vi "Write_To_XML_File.vi"(11 "2D-Array":dbl[][](array[numeric])) -> ()   [LabVIEW 2024]
uses:
  <vilib>/Utility/xml.llb/Read From XML File(string).vi
  <vilib>/Utility/xml.llb/Write to XML File(string).vi
panel:
  in  "Write to XML":bool
  in  "stop":bool
  out "XML Output":string
  out "XML File Path":path
  # "Suppose the 2 D Array is updated at different time. As it is not automated in this VI enter some values\nin the 2D array and press the Write to XML button. Check the output.!!"
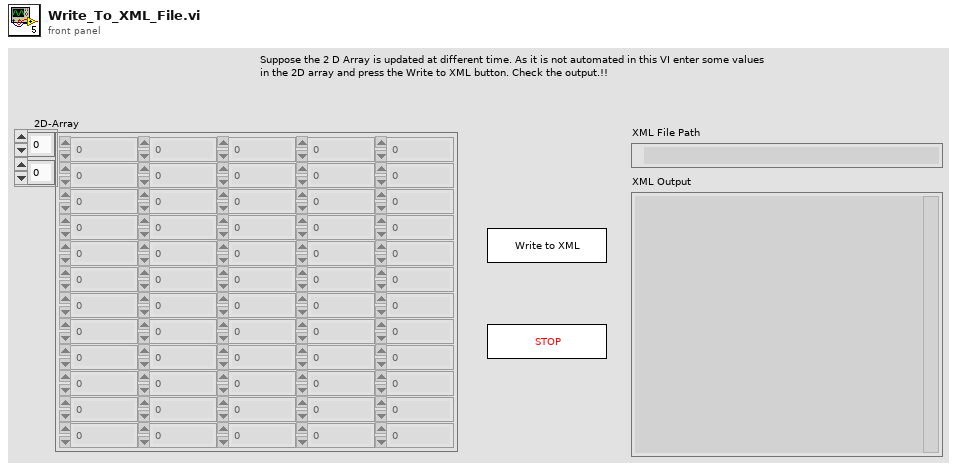
[diagram p1: front panel]
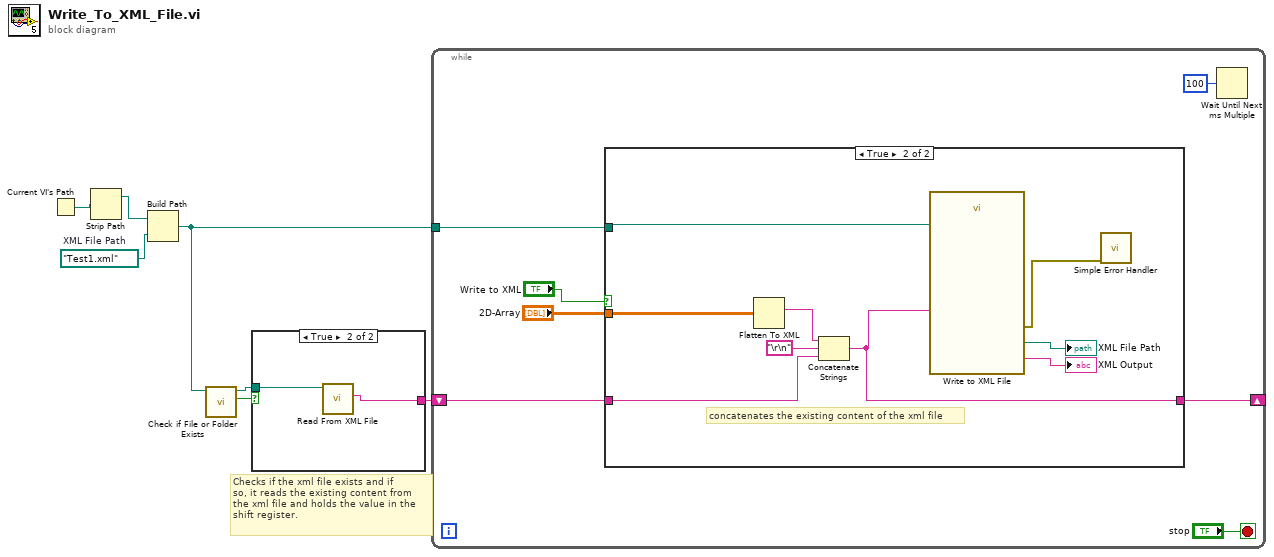
[diagram p0: block diagram]
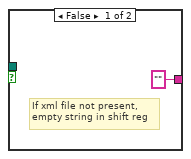
[diagram p2: hidden frame]
diagram:
  w7 = path "Test1.xml"  # XML File Path
  # "Checks if the xml file exists and if\nso, it reads the existing content from\nthe xml file and holds the value in the\nshift register."
  n1 = Current VI's Path() -> (path=w6:path)
  n2 = Strip Path(path=w6) -> (stripped path=w5:path)  [unwired: 1 out]
  n3 = Build Path(base path=w5, name or relative path=w7) -> (appended path=w4:path)
  n4 = call <vilib>:"Check if File or Folder Exists.vi"("path"=w4) -> ("file or folder exists?"=w3:bool, "dup path"=w2:path)  [unwired: 8 in, 1 out]
  n5 = case shown="True" w3 {
    tunnel: w2 -> [_ w10]
    tunnel: ["" ("XML Elements") w9] -> w1
    frame False {
      # "If xml file not present,\nempty string in shift reg"
    }
    frame True {
      n6 = call-poly <vilib>:"Read From XML File.vi"("XML File Path"=w10) -> ("XML Elements"=w9:string)  [unwired: 8 in, 2 out]
    }
  }
  n7 = while {
    tunnel: w4 -> [w17]
    shift-right: [w12] -> _
    shift-left: w1 -> [w13]
    stop <- "stop" stop-if-true
    n8 = case shown="True" "Write to XML" {
      tunnel: w17 -> [_ w24]
      tunnel: "2D-Array" -> [_ w23]
      tunnel: w13 -> [w18 w20]
      tunnel: [w18 w19] -> w12
      frame False {
      }
      frame True {
        # "concatenates the existing content of the xml file"
        n9 = Flatten To XML(6:w23) -> (2:w21:string)
        n10 = Concatenate Strings(w21, "\r\n", w20) -> (w19:string)
        n11 = call-poly <vilib>:"Write to XML File.vi"("XML Input"=w19, "XML File Path"=w24) -> ("error out"=w25:errorcluster, "XML String"=→"XML Output":string, "XML File Path(duplicate)"=→"XML File Path":path)  [unwired: 7 in]
        n12 = call <vilib>:"Simple Error Handler.vi"("error in (no error)"=w25) -> ()  [unwired: 4 in, 5 out]
      }
    }
    n13 = Wait Until Next ms Multiple(millisecond multiple=u32 100) -> ()  [unwired: 1 out]
  }
